vi "Autonomous Independent.vi"() -> ()   [LabVIEW 2014]
doc: "This VI is called when autonomous begins, and will automatically be terminated when autonomous ends. You can carry out timed or sensor driven robot movement independently without needing to return to the caller."
uses:
  <vilib>/Rock Robotics/WPI/RobotDrive/WPI_RobotDriveGetSetRefNum.vi
  <vilib>/Rock Robotics/WPI/RobotDrive/WPI_RobotDriveMecanumDrive_Cartesian.vi
  Desktop/Global 1.vi
  <vilib>/Utility/file.llb/Read From Spreadsheet File (DBL).vi
panel:
  out "Current State":string
  in  "Array":dbl[][](array[numeric])=[[3.0, 0.0], [0.0, 2.0], [-3.0, 0.0], [0.0, -2.0]]
  in  "Mode Select":enum16{"Option 1", "Option 2"}(ring)
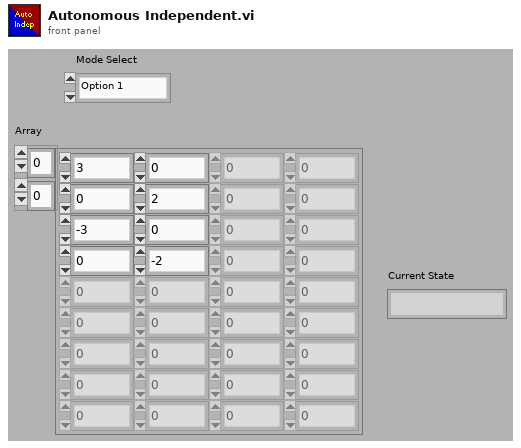
[diagram p1: front panel]
types:
  T1 = typedef "WPI_RobotDriveDevRef.ctl" = cluster{"DevStatus":errorcluster, "Motors[]":T2[], "Square Inputs":bool, "Max Output":dbl}
  T2 = typedef "WPI_MotorControlDeviceRef.ctl" = cluster{"DeviceStatus":errorcluster, "Type":T3, "PWM":cluster{"Controller":T4, "PWM Channel":T5, "DeadBand":T6}, "CAN":cluster{"Device Number":u8, "Control Mode":T7, "Semaphore":T8, "Max Vout":dbl, "TalonSRX Control Mode":T9}, "Invert":bool, "TransformRef":T10, "InvTransformRef":T10}
  T3 = typedef "WPI_MotorControlType.ctl" = enum16{"PWM", "CAN", "CANTalonSRX"}
  T4 = typedef "FPGA_TypedefDigitalModule.ctl" = enum16{"Controller 1"}
  T5 = typedef "FPGA_DIOPWMChannel.ctl" = enum8{"PWM 0", "PWM 1", "PWM 2", "PWM 3", "PWM 4", "PWM 5", "PWM 6", "PWM 7", "PWM 8", "PWM 9", "PWM MXP 0", "PWM MXP 1", "PWM MXP 2", "PWM MXP 3", "PWM MXP 4", "PWM MXP 5", "PWM MXP 6", "PWM MXP 7", "PWM MXP 8", "PWM MXP 9", "Invalid"}
  T6 = typedef "WPI_PWMDeadband.ctl" = cluster{"Name":string, "maxPositivePwm":i32, "minPositivePwm":i32, "centerPwm":i32, "maxNegativePwm":i32, "minNegativePwm":i32, "angularRange":u16}
  T7 = typedef "WPI_CANJaguar_ControlMode.ctl" = enum8{"Percent VBus", "Current", "Speed", "Position", "Voltage"}
  T8 = typedef "Semaphore RefNum" = refnum<k1>
  T9 = typedef "WPI_CANTalonSRX_APIControlMode.ctl" = enum8{"Percent VBus", "Speed", "Position", "Slave", "Unchanged / Invalid"}
  T10 = typedef "WPI_PWMTransform_ConPane.ctl" = refnum<vi>
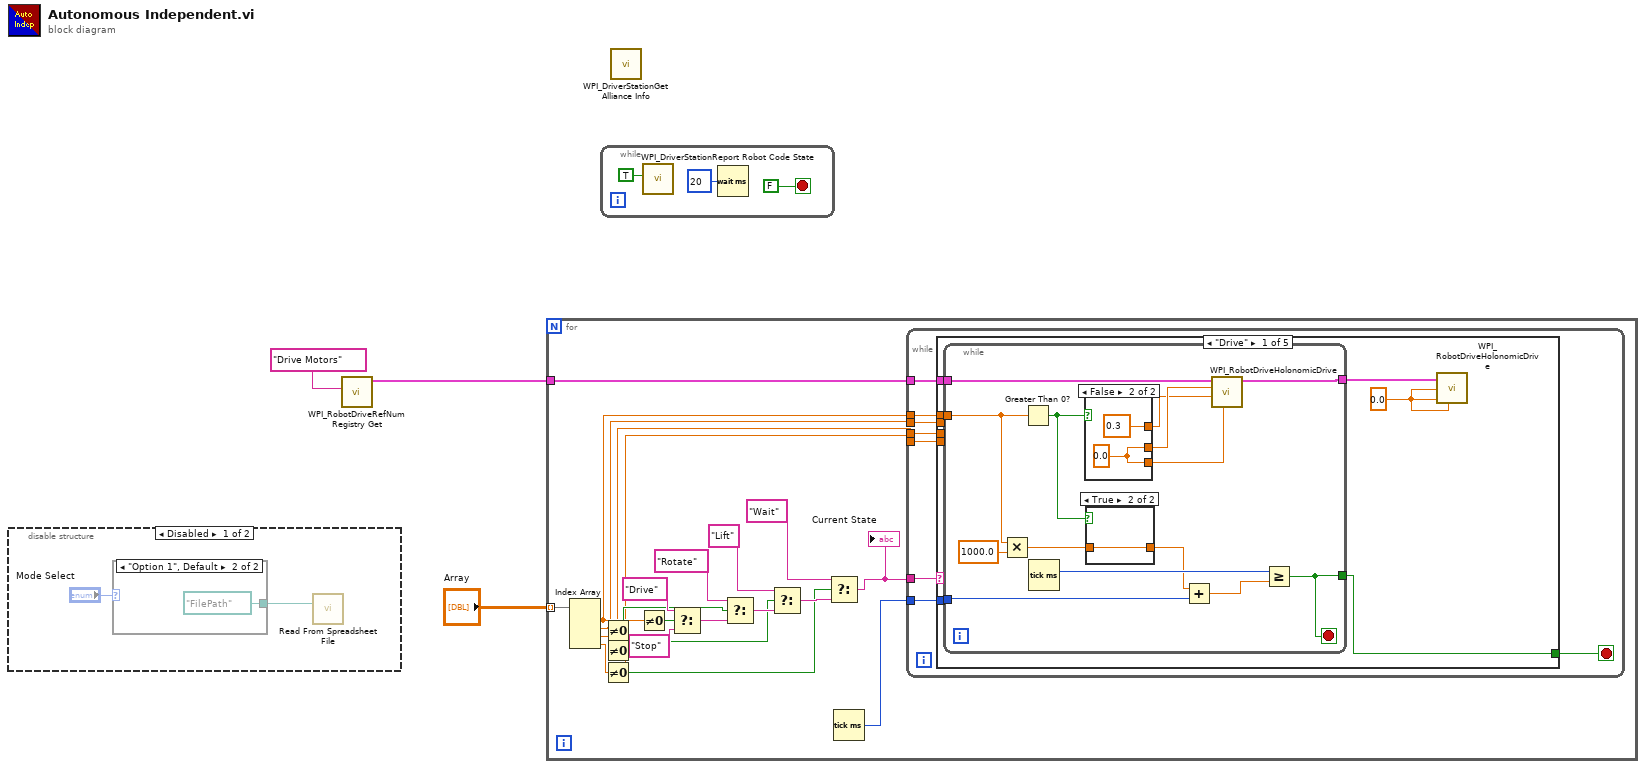
[diagram p0: block diagram]
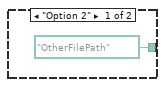
[diagram p2: hidden frame]
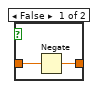
[diagram p4: hidden frame]
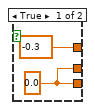
[diagram p5: hidden frame]
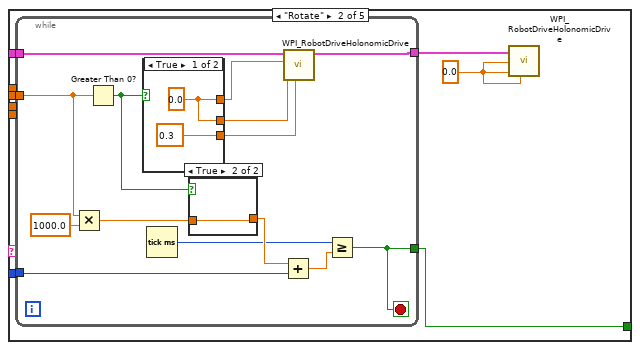
[diagram p6: hidden frame]
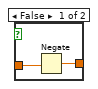
[diagram p7: hidden frame]
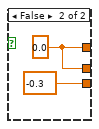
[diagram p8: hidden frame]
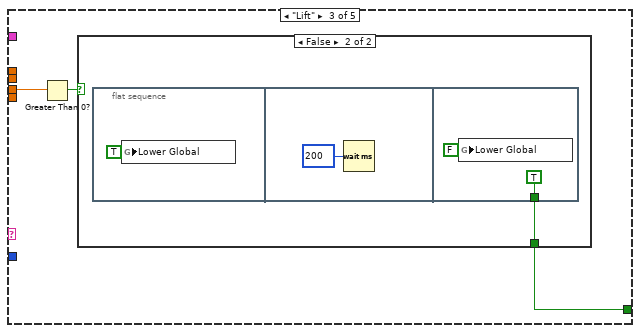
[diagram p9: hidden frame]
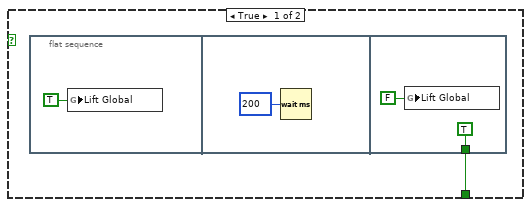
[diagram p10: hidden frame]
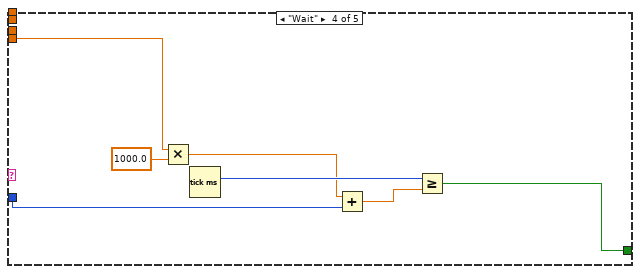
[diagram p11: hidden frame]
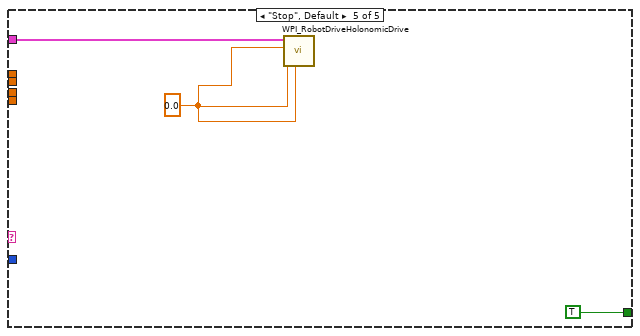
[diagram p12: hidden frame]
diagram:
  n1 = disable-structure shown="Disabled" {
    frame Disabled {
      n2 = case shown="\"Option 1\", Default" "Mode Select" {
        tunnel: [path "OtherFilePath" ("file path (dialog if empty)") path "FilePath" ("file path (dialog if empty)")] -> w5
        frame "Option 2" {
        }
        frame "Option 1", Default {
        }
      }
      n3 = call-poly <vilib>:"Read From Spreadsheet File.vi"("file path (dialog if empty)"=w5) -> ()  [unwired: 6 in, 5 out]
    }
    frame Enabled {
    }
  }
  n4 = call <vilib>:"WPI_RobotDriveRefNum Registry Get.vi"("refnum name"="Drive Motors") -> ("RobotDriveDevRef"=w2:T1)  [unwired: 9 in, 1 out]
  n5 = for {
    tunnel: w2 -> [w15]
    tunnel: "Array" -> [w8] mode=indexing
    n6 = Index Array(array=w8) -> (element #1=w14:dbl, element #2=w12:dbl, element #3=w11:dbl, element #4=w10:dbl)  [unwired: 4 in]
    n7 = Not Equal To 0?(x=w12) -> (x != 0?=w18:bool)
    n8 = Not Equal To 0?(x=w11) -> (x != 0?=w17:bool)
    n9 = Not Equal To 0?(x=w10) -> (x != 0?=w16:bool)
    n10 = Not Equal To 0?(x=w14) -> (x != 0?=w27:bool)
    n11 = Select(t="Drive", s=w27, f="Stop") -> (s? t:f=w24:string)
    n12 = Select(t="Rotate", s=w18, f=w24) -> (s? t:f=w22:string)
    n13 = Select(t="Lift", s=w17, f=w22) -> (s? t:f=w20:string)
    n14 = Select(t="Wait", s=w16, f=w20) -> (s? t:f=w9:string)
    "Current State" <- w9
    n15 = Tick Count (ms)() -> (millisecond timer value=w13:u32)
    n16 = while {
      tunnel: w9 -> [w35]
      tunnel: w15 -> [w34]
      tunnel: w14 -> [w33]
      tunnel: w13 -> [w32]
      tunnel: w12 -> [w31]
      tunnel: w11 -> [w30]
      tunnel: w10 -> [w29]
      stop <- w28 stop-if-true
      n17 = case shown="\"Drive\"" w35 {
        tunnel: w34 -> [w40 w67 _ _ w112]
        tunnel: w33 -> [w38 _ _ _ _]
        tunnel: w32 -> [w37 w65 _ w105 _]
        tunnel: w31 -> [_ w64 _ _ _]
        tunnel: w30 -> [_ _ w92 _ _]
        tunnel: w29 -> [_ _ _ w104 _]
        tunnel: [w36 w63 w90 w103 TRUE] -> w28
        frame "Drive" {
          w41 = 0.0 ("X")
          n18 = while {
            tunnel: w40 -> [w54]
            tunnel: [w53] -> w39
            tunnel: w38 -> [w52]
            tunnel: w37 -> [w49]
            tunnel: [w47] -> w36
            stop <- w47 stop-if-true
            n19 = Multiply(x=w52, y=1000.0) -> (x*y=w45:dbl)
            n20 = Greater Than 0?(x=w52) -> (x > 0?=w46:bool)
            n21 = Tick Count (ms)() -> (millisecond timer value=w50:u32)
            n22 = case shown="False" w46 {
              tunnel: [-0.3 ("X") 0.3 ("X")] -> w42
              tunnel: [w59 w61] -> w43
              tunnel: [w59 w61] -> w55
              frame True {
                w59 = 0.0 ("Rotation")
              }
              frame False {
                w61 = 0.0 ("Rotation")
              }
            }
            n23 = case shown="True" w46 {
              tunnel: w45 -> [w56 w58]
              tunnel: [w57 w58] -> w44
              frame False {
                n24 = Negate(x=w56) -> (-x=w57:dbl)
              }
              frame True {
              }
            }
            n25 = Add(x=w44, y=w49) -> (x+y=w48:dbl)
            n26 = call-poly <vilib>:"WPI_RobotDriveHolonomicDrive.vi"("Rotation"=w55, "Y"=w42, "X"=w43, "RobotDriveDevRef"=w54) -> ("RobotDriveDevRef"=w53:T1)  [unwired: 5 in, 2 out]
            n27 = Greater Or Equal?(x=w50, y=w48) -> (x >= y?=w47:bool)
          }
          n28 = call-poly <vilib>:"WPI_RobotDriveHolonomicDrive.vi"("Rotation"=w41, "Y"=w41, "X"=w41, "RobotDriveDevRef"=w39) -> ()  [unwired: 5 in, 3 out]
        }
        frame "Rotate" {
          w68 = 0.0 ("X")
          n29 = while {
            tunnel: w67 -> [w80]
            tunnel: [w79] -> w66
            tunnel: w65 -> [w77]
            tunnel: w64 -> [w75]
            tunnel: [w74] -> w63
            stop <- w74 stop-if-true
            n30 = Multiply(x=w75, y=1000.0) -> (x*y=w72:dbl)
            n31 = Greater Than 0?(x=w75) -> (x > 0?=w73:bool)
            n32 = case shown="True" w73 {
              tunnel: [w86 w88] -> w76
              tunnel: [w86 w88] -> w82
              tunnel: [0.3 ("Rotation") -0.3 ("Rotation")] -> w81
              frame True {
                w86 = 0.0 ("X")
              }
              frame False {
                w88 = 0.0 ("X")
              }
            }
            n33 = Tick Count (ms)() -> (millisecond timer value=w70:u32)
            n34 = case shown="True" w73 {
              tunnel: [w84 w85] -> w71
              tunnel: w72 -> [w83 w85]
              frame False {
                n35 = Negate(x=w83) -> (-x=w84:dbl)
              }
              frame True {
              }
            }
            n36 = Add(x=w71, y=w77) -> (x+y=w69:dbl)
            n37 = call-poly <vilib>:"WPI_RobotDriveHolonomicDrive.vi"("Rotation"=w81, "Y"=w82, "X"=w76, "RobotDriveDevRef"=w80) -> ("RobotDriveDevRef"=w79:T1)  [unwired: 5 in, 2 out]
            n38 = Greater Or Equal?(x=w70, y=w69) -> (x >= y?=w74:bool)
          }
          n39 = call-poly <vilib>:"WPI_RobotDriveHolonomicDrive.vi"("Rotation"=w68, "Y"=w68, "X"=w68, "RobotDriveDevRef"=w66) -> ()  [unwired: 5 in, 3 out]
        }
        frame "Lift" {
          n40 = Greater Than 0?(x=w92) -> (x > 0?=w91:bool)
          n41 = case shown="False" w91 {
            tunnel: [w93 w98] -> w90
            frame True {
              n42 = flat-sequence {
                tunnel: [TRUE] -> w93
                frame #0 {
                  n43 = global write "Global 1.vi" "Lift Global"(TRUE ("Lift Global")) -> ()
                }
                frame #1 {
                  n44 = Wait (ms)(milliseconds to wait=u32 200) -> ()  [unwired: 1 out]
                }
                frame #2 {
                  n45 = global write "Global 1.vi" "Lift Global"(FALSE ("Lift Global")) -> ()
                }
              }
            }
            frame False {
              n46 = flat-sequence {
                tunnel: [TRUE] -> w98
                frame #0 {
                  n47 = global write "Global 1.vi" "Lower Global"(TRUE ("Lift Global")) -> ()
                }
                frame #1 {
                  n48 = Wait (ms)(milliseconds to wait=u32 200) -> ()  [unwired: 1 out]
                }
                frame #2 {
                  n49 = global write "Global 1.vi" "Lower Global"(FALSE ("Lift Global")) -> ()
                }
              }
            }
          }
        }
        frame "Wait" {
          n50 = Multiply(x=w104, y=1000.0) -> (x*y=w106:dbl)
          n51 = Tick Count (ms)() -> (millisecond timer value=w108:u32)
          n52 = Add(x=w106, y=w105) -> (x+y=w109:dbl)
          n53 = Greater Or Equal?(x=w108, y=w109) -> (x >= y?=w103:bool)
        }
        frame "Stop", Default {
          w111 = 0.0 ("Rotation")
          n54 = call-poly <vilib>:"WPI_RobotDriveHolonomicDrive.vi"("Rotation"=w111, "Y"=w111, "X"=w111, "RobotDriveDevRef"=w112) -> ()  [unwired: 5 in, 3 out]
        }
      }
    }
  }
  n55 = while {
    stop <- FALSE stop-if-true
    n56 = call <vilib>:"WPI_DriverStationReport Robot Code State.vi"("Autonomous"=TRUE) -> ()  [unwired: 10 in, 1 out]
    n57 = Wait (ms)(milliseconds to wait=u32 20) -> ()  [unwired: 1 out]
  }
  n58 = call <vilib>:"WPI_DriverStationGet Alliance Info.vi"() -> ()  [unwired: 12 out]
